vi "MAIN prod-cons combined v1.vi"() -> ()   [LabVIEW 2012]
doc: "Use this template to build a producer/consumer design pattern. Use this template when you need to execute a process, such as data analysis, when a data source, such as a triggered acquisition, produces data at an uneven rate and you need to execute the process when the data becomes available."
uses:
  <vilib>/Instr/_visa.llb/VISA Configure Serial Port (Instr).vi
panel:
  in  "analysis of text file on/off":bool
  in  "stop reading the text file":bool
  in  "INPUT:\non = serial\noff = text file":bool
  in  "XON Character":u8=17 format="%.0x"
  in  "XOFF Character":u8=19 format="%.0x"
  in  "flow control":u16(ring) items=["None"=0, "XON/XOFF"=1, "RTS/CTS"=2, "DTR/DSR"=4]
  in  "End write with termination character?":bool=TRUE
  in  "Input\nbuffer size":u32=4096
  in  "bytes to read":u32=1000
  out "actual bytes read":u32
  in  "write":bool=TRUE
  in  "read":bool=TRUE
  in  "stop 2":bool
  in  "string to write":string="*IDN?"
  in  "termination char\n(0xA = '\\n' = LF)":u8=10 format="%.0x"
  in  "End read on termination character?":bool=TRUE
  in  "timeout (ms)":u32=10000
  in  "stop bits":u16(ring)=10 items=["1.0"=10, "1.5"=15, "2.0"=20]
  in  "parity":u16(ring) items=["None", "Odd", "Even", "Mark", "Space"]
  in  "data bits":u16=8 min=5 max=8 step=1
  in  "VISA resource name":refnum<visa-resource-name>="COM1"
  in  "baud rate":u32=9600
  out "Camera 1":picture
  out "Temperature":waveform(i64)[](graph)
  out "Pressure":waveform(i64)[](graph)
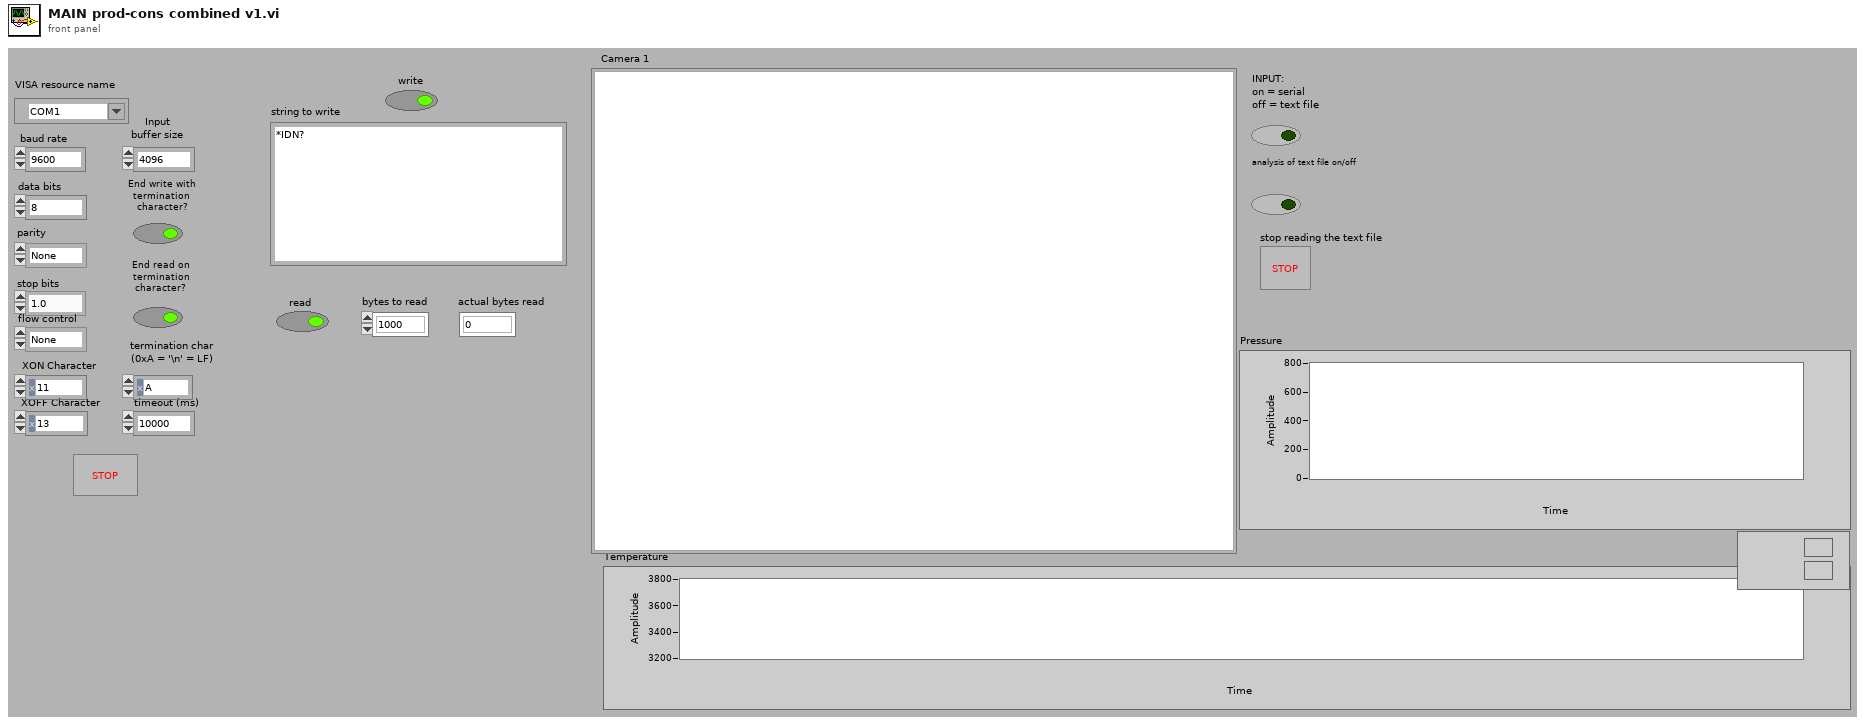
[diagram p1: front panel]
types:
  T1 = enum16{"open", "replace", "create", "open or create", "replace or create", "replace or create with confirmation"}
  T2 = cluster{"left":i16, "top":i16, "right":i16, "bottom":i16}
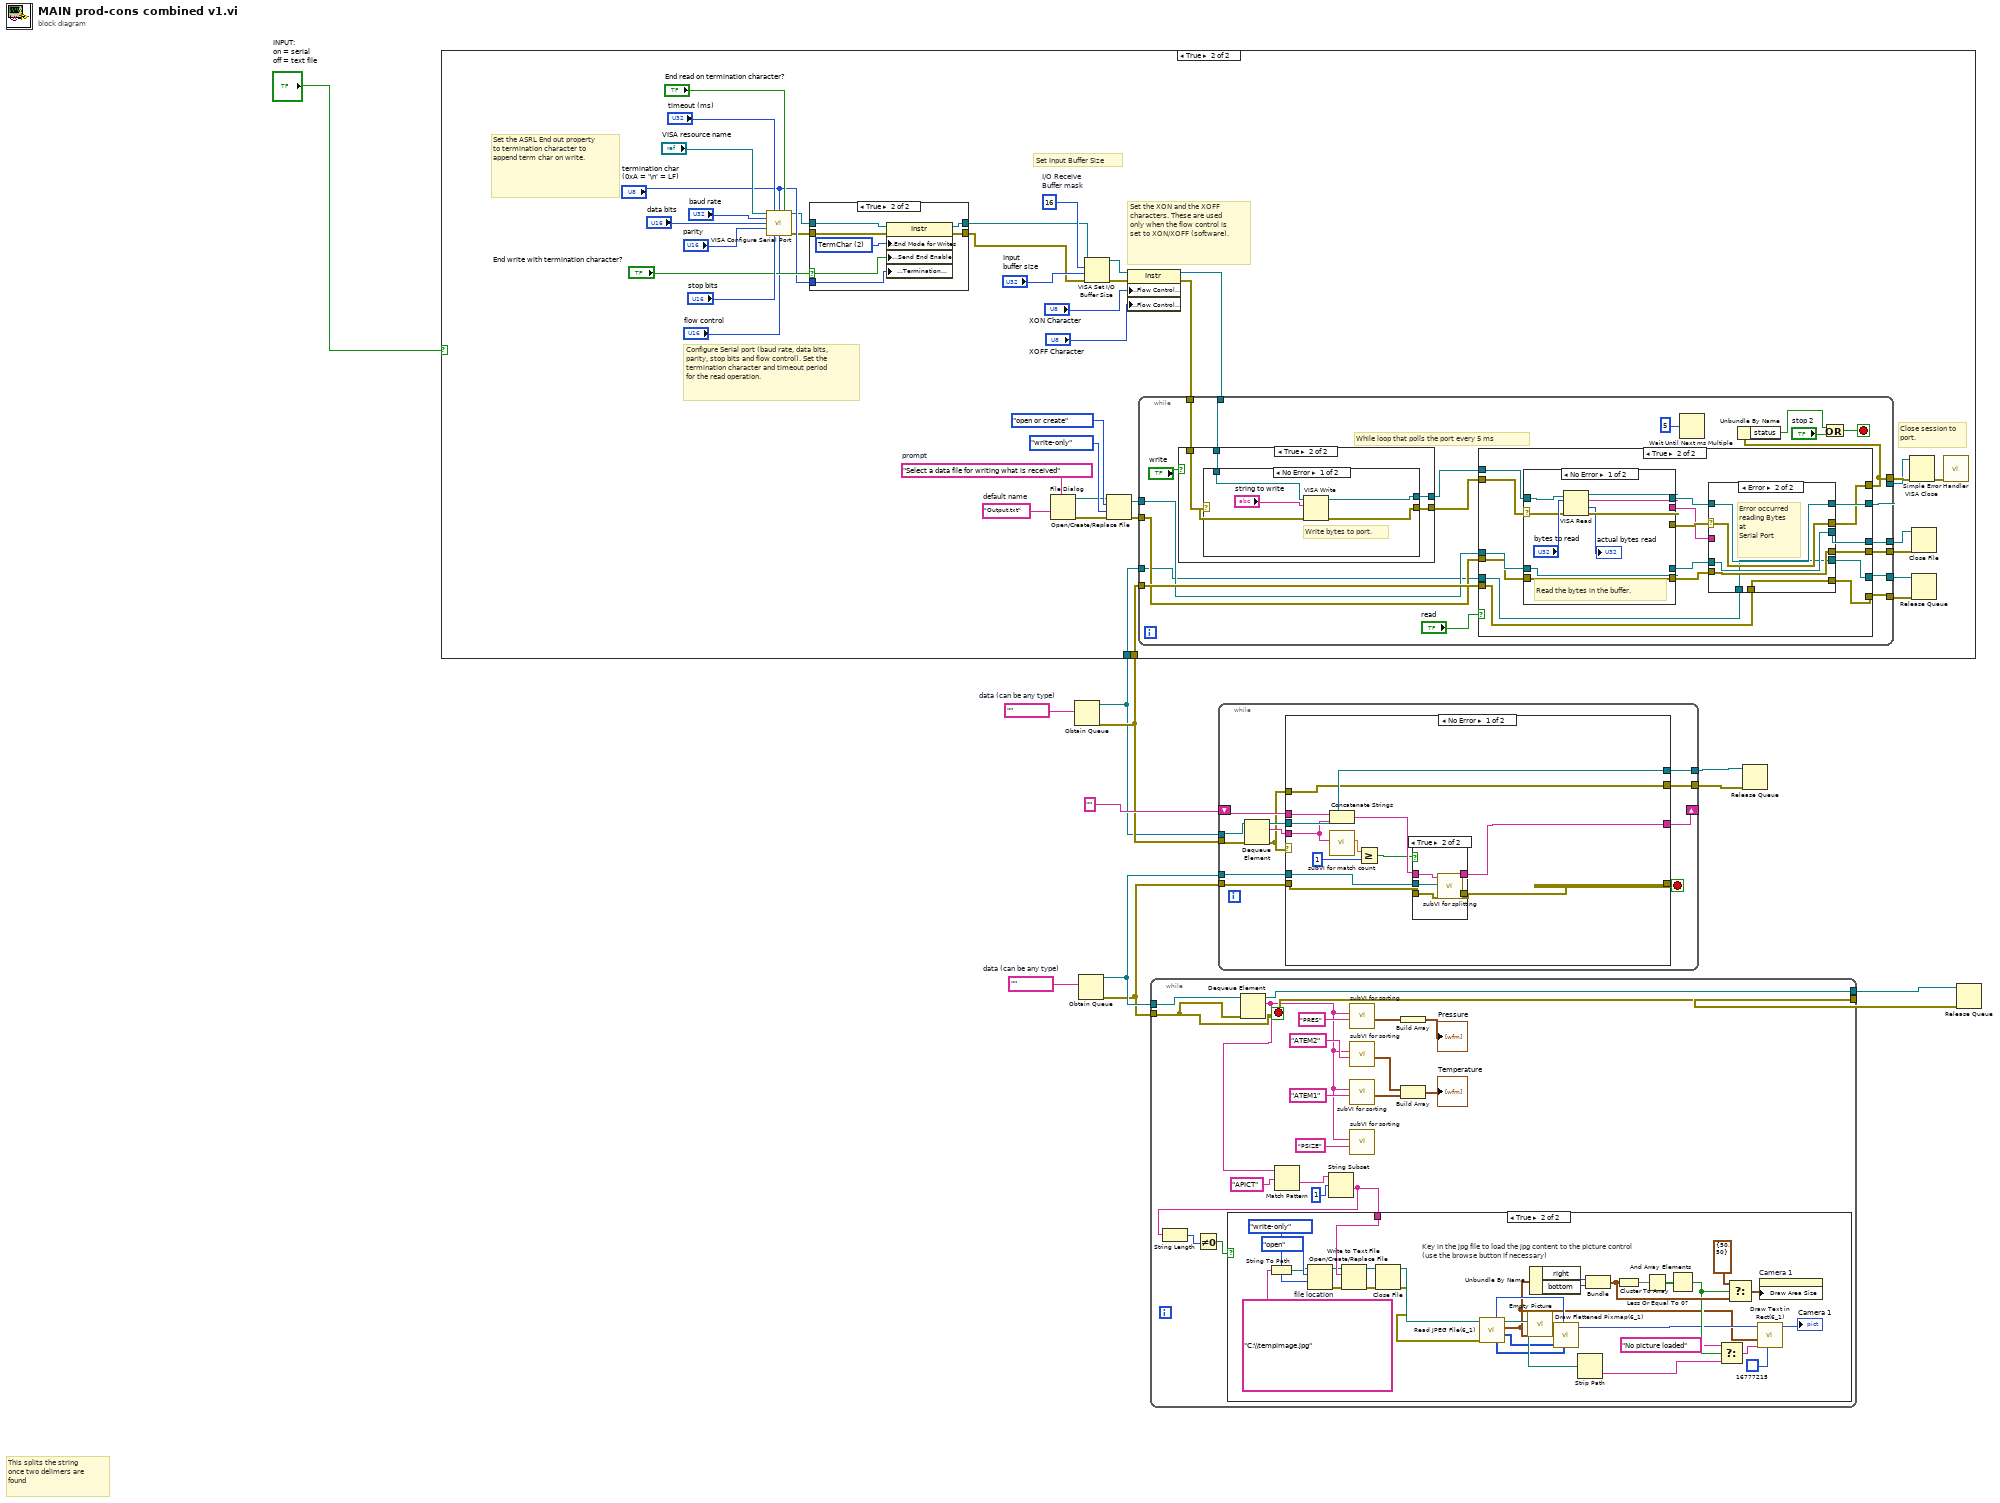
[diagram p0: block diagram]
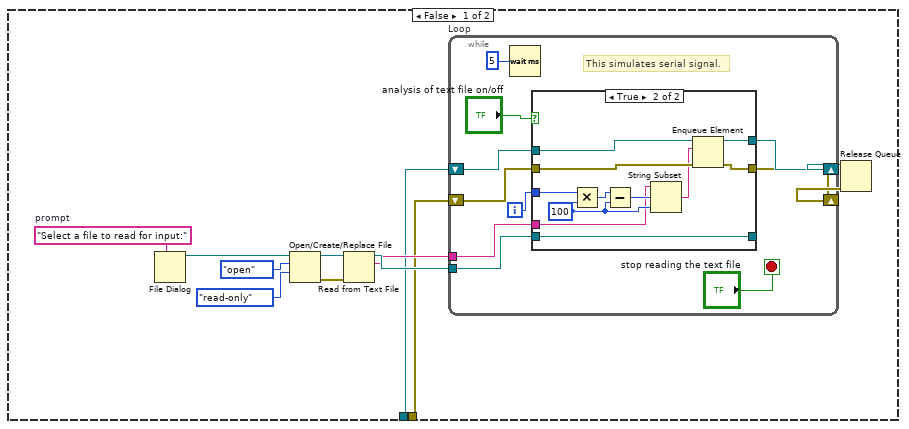
[diagram p2: hidden frame]
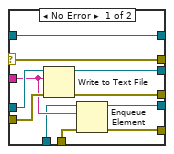
[diagram p8: hidden frame]
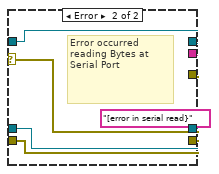
[diagram p9: hidden frame]
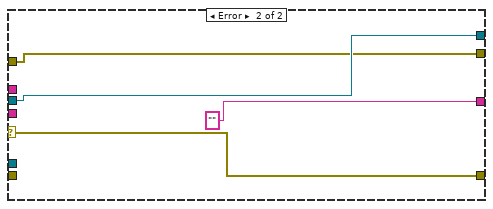
[diagram p12: hidden frame]
diagram:
  w11 = ""  # data (can be any type)
  w12 = ""  # data (can be any type)
  # "This splits the string once two delimers are found"
  n1 = Obtain Queue(element data type=w12) -> (queue out=w2:refnum<queue>, error out=w3:errorcluster)  [unwired: 4 in, 1 out]
  n2 = case shown="True" "INPUT:\non = serial\noff = text file" {
    tunnel: w3 -> [w14 w50]
    tunnel: w2 -> [w13 w49]
    frame False {
      w18 = "Select a file to read for input:"  # prompt
      n3 = File Dialog(7:w18) -> (3:w16:path)  [unwired: 1 in, 8 out]
      n4 = Open/Create/Replace File(file path (use dialog)=w16, operation (0:open)=T1."open", access (0:read/write)=enum16{"read/write", "read-only", "write-only"}."read-only") -> (refnum out=w21:refnum<file>, error out=w22:errorcluster)  [unwired: 1 in, 3 out]
      n5 = Read from Text File(file (use dialog)=w21, error in=w22) -> (refnum out=w17:refnum<file>, text=w15:string)  [unwired: 1 in, 3 out]
      n6 = while "Loop" {
        shift-right: [w26] -> w23
        shift-left: w14 -> [w32]
        shift-right: [w27] -> w24
        shift-left: w13 -> [w33]
        tunnel: w15 -> [w31]
        tunnel: w17 -> [w30]
        i -> [w29]
        stop <- "stop reading the text file" stop-if-true
        # "This simulates serial signal."
        n7 = Wait (ms)(milliseconds to wait=u32 5) -> ()  [unwired: 1 out]
        n8 = case shown="True" "analysis of text file on/off" {
          tunnel: w30 -> [w37 w45]
          tunnel: [w37 w45] -> _
          tunnel: w31 -> [_ w43]
          tunnel: w33 -> [w35 w41]
          tunnel: w32 -> [w36 w40]
          tunnel: w29 -> [_ w44]
          tunnel: [w35 w42] -> w27
          tunnel: [w36 w39] -> w26
          frame False {
          }
          frame True {
            w46 = 100
            n9 = Multiply(x=w44, y=w46) -> (x*y=w48:i32)
            n10 = Subtract(x=w48, y=w46) -> (x-y=w47:i32)
            n11 = String Subset(string=w43, offset (0)=w47, length (rest)=w46) -> (substring=w38:string)
            n12 = Enqueue Element(queue=w41, element=w38, error in (no error)=w40) -> (queue out=w42:refnum<queue>, error out=w39:errorcluster)  [unwired: 1 in, 1 out]
          }
        }
      }
      n13 = Release Queue(queue=w24, error in (no error)=w23) -> ()  [unwired: 1 in, 3 out]
    }
    frame True {
      w59 = "Output.txt"  # default name
      w60 = "Select a data file for writing what is received"  # prompt
      w80 = u16 16  # I/O Receive Buffer mask
      # "Set the XON and the XOFF characters. These are used only when the flow control is set to XON/XOFF (software)."
      # "Configure Serial port (baud rate, data bits, parity, stop bits and flow control). Set the termination character and timeout period for the read operation."
      # "Set Input Buffer Size"
      # "Set the ASRL End out property to termination character to append term char on write."
      # "Close session to port."
      n14 = call-poly "VISA Configure Serial Port"("VISA resource name"="VISA resource name", "timeout (10sec)"="timeout (ms)", "termination char\n(0xA = '\\n' = LF)"="termination char\n(0xA = '\\n' = LF)", "Enable Termination\nChar (T)"="End read on termination character?", "baud rate (9600)"="baud rate", "data bits (8)"="data bits", "parity (0:none)"="parity", "stop bits (10: 1 bit)"="stop bits", "flow control (0:none)"="flow control") -> ("VISA resource name out"=w66:refnum<visa-resource-name>, "error out"=w69:errorcluster)  [unwired: 1 in, 4 out]
      n15 = case shown="True" "End write with termination character?" {
        selector: "End write with termination character?" -> [_ w90]
        tunnel: w66 -> [w88 w96]
        tunnel: w69 -> [w89 w95]
        tunnel: [w88 w94] -> w67
        tunnel: [w89 w93] -> w68
        tunnel: "termination char\n(0xA = '\\n' = LF)" -> [_ w91]
        frame False {
        }
        frame True {
          w92 = u16 2 items=["None", "LastBit", "TermChar", "Break"] ("Serial Settings:Serial End Mode for Writes")
          n16 = property class="Instr"(reference=w96, error in=w95, "Serial Settings:End Mode for Writes"=w92, "Message Based Settings:Send End Enable"=w90, "Message Based Settings:Termination Character"=w91) -> (reference out=w94:refnum<visa-resource-name>, error out=w93:errorcluster)
        }
      }
      n17 = File Dialog(7:w60, 9:w59) -> (0:w61:errorcluster, 3:w58:path)  [unwired: 1 in, 6 out]
      n18 = VISA Set I/O Buffer Size(VISA resource name=w67, mask (16)=w80, size (4096)="Input\nbuffer size", error in (no error)=w68) -> (VISA resource name out=w75:refnum<visa-resource-name>, error out=w74:errorcluster)
      n19 = Open/Create/Replace File(file path (use dialog)=w58, error in=w61, operation (0:open)=T1."open or create", access (0:read/write)=enum16{"read/write", "read-only", "write-only"}."write-only") -> (refnum out=w54:refnum<file>, error out=w55:errorcluster)  [unwired: 3 out]
      n20 = property class="Instr"(reference=w75, error in=w74, "Serial Settings:Flow Control XON Character"="XON Character", "Serial Settings:Flow Control XOFF Character"="XOFF Character") -> (reference out=w65:refnum<visa-resource-name>, error out=w71:errorcluster)
      n21 = while {
        tunnel: w71 -> [w97]
        tunnel: w65 -> [w112]
        tunnel: [w104] -> w51
        tunnel: [w100] -> w64
        tunnel: [w109] -> w57
        tunnel: [w108] -> w56
        tunnel: w55 -> [w103]
        tunnel: w54 -> [w102]
        tunnel: [w107] -> w53
        tunnel: [w106] -> w52
        tunnel: w49 -> [w101]
        tunnel: w50 -> [w105]
        stop <- w111 stop-if-true
        # "While loop that polls the port every 5 ms"
        n22 = case shown="True" "write" {
          tunnel: [w118 w122] -> w99
          tunnel: [w117 w121] -> w98
          tunnel: w112 -> [w118 w120]
          tunnel: w97 -> [w117 w119]
          frame False {
          }
          frame True {
            n23 = case shown="No Error" w119 {
              selector: w119 -> [w123 w129]
              tunnel: [w127 w128] -> w122
              tunnel: [w126 w129] -> w121
              tunnel: w120 -> [w124 w128]
              frame No Error {
                # "Write bytes to port."
                n24 = VISA Write(VISA resource name=w124, write buffer="string to write", error in (no error)=w123) -> (VISA resource name out=w127:refnum<visa-resource-name>, error out=w126:errorcluster)  [unwired: 1 out]
              }
              frame Error {
              }
            }
          }
        }
        n25 = case shown="True" "read" {
          tunnel: w98 -> [w134 w152]
          tunnel: w99 -> [w135 w151]
          tunnel: [w134 w141] -> w100
          tunnel: [w135 w143] -> w104
          tunnel: [w132 w145] -> w109
          tunnel: [w133 w147] -> w108
          tunnel: w102 -> [w133 w150]
          tunnel: w103 -> [w132 w149]
          tunnel: [w130 w138] -> w107
          tunnel: [w131 w139] -> w106
          tunnel: w101 -> [w131 w137]
          tunnel: w105 -> [w130 w136]
          frame False {
          }
          frame True {
            n26 = case "Read bytes from port." shown="No Error" w152 {
              selector: w152 -> [w174 w182]
              tunnel: [w177 w182] -> w142
              tunnel: [w178 w183] -> w144
              tunnel: w151 -> [w175 w183]
              tunnel: [w172 w180] -> w146
              tunnel: [w171 w181] -> w148
              tunnel: w150 -> [w171 w181]
              tunnel: w149 -> [w172 w180]
              tunnel: [w170 "[error in serial read}" ("read buffer")] -> w140
              frame No Error {
                # "Read the bytes in the buffer."
                n27 = VISA Read(VISA resource name=w175, byte count="bytes to read", error in (no error)=w174) -> (VISA resource name out=w178:refnum<visa-resource-name>, read buffer=w170:string, return count=→"actual bytes read":u32, error out=w177:errorcluster)
              }
              frame Error {
                # "Error occurred \nreading Bytes at \nSerial Port"
              }
            }
            n28 = case "Read bytes from port." shown="Error" w142 {
              selector: w142 -> [w163 w166]
              tunnel: [w163 w166] -> w141
              tunnel: w148 -> [w159 w169]
              tunnel: [w158 w169] -> w147
              tunnel: w146 -> [w161 w168]
              tunnel: [w160 w168] -> w145
              tunnel: w144 -> [w162 w167]
              tunnel: [w162 w167] -> w143
              tunnel: w140 -> [w155 _]
              tunnel: [w157 w165] -> w139
              tunnel: [w156 w164] -> w138
              tunnel: w137 -> [w154 w165]
              tunnel: w136 -> [w153 w164]
              frame No Error {
                n29 = Write to Text File(file (use dialog)=w159, text=w155, error in=w161) -> (refnum out=w158:refnum<file>, error out=w160:errorcluster)  [unwired: 1 in, 1 out]
                n30 = Enqueue Element(queue=w154, element=w155, error in (no error)=w153) -> (queue out=w157:refnum<queue>, error out=w156:errorcluster)  [unwired: 1 in, 1 out]
              }
              frame Error {
                # "Error occurred \nreading Bytes at \nSerial Port"
              }
            }
          }
        }
        n31 = Wait Until Next ms Multiple(millisecond multiple=u32 5) -> ()  [unwired: 1 out]
        n32 = Unbundle By Name(w100) -> ("status"=w114:bool)
        n33 = Or(x=w114, y="stop 2") -> (x .or. y?=w111:bool)
      }
      n34 = VISA Close(VISA resource name=w51, error in (no error)=w64) -> (error out=w85:errorcluster)
      n35 = Close File(refnum=w56, error in=w57) -> ()  [unwired: 2 out]
      n36 = Release Queue(queue=w52, error in (no error)=w53) -> ()  [unwired: 1 in, 3 out]
      n37 = call <vilib>:"Simple Error Handler.vi"("error in (no error)"=w85) -> ()  [unwired: 1 in, 8 out]
    }
  }
  n38 = Obtain Queue(element data type=w11) -> (queue out=w10:refnum<queue>, error out=w9:errorcluster)  [unwired: 4 in, 1 out]
  n39 = while {
    tunnel: w10 -> [w202]
    tunnel: w9 -> [w201]
    tunnel: [w192] -> w6
    tunnel: [w191] -> w5
    stop <- w201 stop-if-true
    n40 = Dequeue Element(queue=w202, error in (no error)=w201) -> (queue out=w192:refnum<queue>, element=w190:string, error out=w191:errorcluster)  [unwired: 1 in, 1 out]
    n41 = Match Pattern(string=w190, regular expression="APICT" ("identifier")) -> (after substring=w188:string)  [unwired: 1 in, 3 out]
    n42 = String Subset(string=w188, offset (0)=1) -> (substring=w186:string)  [unwired: 1 in]
    n43 = String Length(string=w186) -> (length=w185:i32)
    n44 = Not Equal To 0?(x=w185) -> (x != 0?=w184:bool)
    n45 = case shown="True" w184 {
      tunnel: w186 -> [_ w234]
      frame False {
      }
      frame True {
        w226 = "C:\\tempimage.jpg"  # file location
        # "Key in the jpg file to load the jpg content to the picture control\n(use the browse button if necessary)"
        n46 = String To Path(string=w226) -> (path=w227:path)
        n47 = Open/Create/Replace File(file path (use dialog)=w227, operation (0:open)=T1."open", access (0:read/write)=enum16{"read/write", "read-only", "write-only"}."write-only") -> (refnum out=w229:refnum<file>, error out=w228:errorcluster)  [unwired: 3 in, 1 out]
        n48 = Write to Text File(file (use dialog)=w229, text=w234, error in=w228) -> (refnum out=w233:refnum<file>, error out=w232:errorcluster)  [unwired: 1 in, 1 out]
        n49 = Close File(refnum=w233, error in=w232) -> (path=w205:path, error out=w204:errorcluster)
        n50 = call <vilib>:"Read JPEG File(6_1).vi"("error in (no error)"=w204, "path to JPEG file"=w205) -> ("flattened image data"=w206:u8[], "rect"=w211:T2, "path"=w213:path, "colorTable"=w210:u32[], "depth"=w225:u8)  [unwired: 4 in, 1 out]
        n51 = call "Empty Picture"() -> ("empty picture"=w224:picture)
        n52 = Unbundle By Name(w211) -> ("right"=w222:i16, "bottom"=w223:i16)
        n53 = call <vilib>:"Draw Flattened Pixmap(6_1).vi"("picture"=w224, "bit depth(8)"=w225, "rect"=w211, "flattened pixmap data"=w206, "color table"=w210) -> ("new picture"=w214:picture)  [unwired: 4 in]
        n54 = Strip Path(path=w213) -> (name=w212:string)  [unwired: 1 out]
        n55 = Bundle("right"=w222, "bottom"=w223) -> (w219:cluster{"right":i16, "bottom":i16})  [unwired: 1 in]
        n56 = Cluster To Array(cluster=w219) -> (array=w221:i16[])
        n57 = Less Or Equal To 0?(x=w221) -> (x <= 0?=w220:bool[])
        n58 = And Array Elements(Boolean array=w220) -> (logical AND=w218:bool)
        n59 = Select(t="No picture loaded", s=w218, f=w212) -> (s? t:f=w216:string)
        n60 = Select(t=cluster{"Width":u32, "Height":u32} {"Width"=50, "Height"=50} ("Draw Area Size"), s=w218, f=w219) -> (s? t:f=w208:cluster{"Width":u32, "Height":u32})
        n61 = call <vilib>:"Draw Text in Rect(6_1).vi"("text color(black)"=u32 16777215, "text"=w216, "rect"=w211, "picture"=w214) -> ("new picture"=→"Camera 1":picture)  [unwired: 7 in]
        n62 = property on="Camera 1" class="Pict"("Draw Area Size"=w208) -> ()  [unwired: 2 in, 2 out]
      }
    }
    n63 = call "subVI for sorting.vi"("identifier"="PRES", "string"=w190) -> ("output"=w199:waveform(i64))  [unwired: 7 in, 2 out]
    n64 = call "subVI for sorting.vi"("identifier"="ATEM2", "string"=w190) -> ("output"=w196:waveform(i64))  [unwired: 7 in, 2 out]
    n65 = call "subVI for sorting.vi"("identifier"="ATEM1", "string"=w190) -> ("output"=w194:waveform(i64))  [unwired: 7 in, 2 out]
    n66 = call "subVI for sorting.vi"("identifier"="PSIZE", "string"=w190) -> ()  [unwired: 7 in, 3 out]
    n67 = Build Array(w199) -> (→"Pressure":waveform(i64)[])
    n68 = Build Array(w196, w194) -> (→"Temperature":waveform(i64)[])
  }
  n69 = while {
    tunnel: w2 -> [w246]
    tunnel: w3 -> [w244]
    shift-right: [w243] -> _
    shift-left: "" ("substring") -> [w242]
    tunnel: w9 -> [w241]
    tunnel: w10 -> [w240]
    tunnel: [w237] -> w8
    tunnel: [w236] -> w7
    stop <- w239 stop-if-true
    n70 = Dequeue Element(queue=w246, error in (no error)=w244) -> (queue out=w238:refnum<queue>, element=w245:string, error out=w235:errorcluster)  [unwired: 1 in, 1 out]
    n71 = case shown="No Error" w235 {
      selector: w235 -> [_ w268]
      tunnel: w245 -> [w248 _]
      tunnel: [w252 ""] -> w243
      tunnel: w242 -> [w250 _]
      tunnel: w241 -> [w257 _]
      tunnel: w240 -> [w256 _]
      tunnel: [w255 w268] -> w239
      tunnel: w238 -> [w254 w267]
      tunnel: [w254 w267] -> w237
      tunnel: w235 -> [w253 w266]
      tunnel: [w253 w266] -> w236
      frame No Error {
        n72 = Concatenate Strings(w250, w248) -> (w258:string)
        n73 = call "subVI for match count.vi"("String"=w248) -> ("Number of matches for \\n"=w247:dbl)  [unwired: 10 in]
        n74 = Greater Or Equal?(x=w247, y=1 ("x")) -> (x >= y?=w249:bool)
        n75 = case shown="True" w249 {
          tunnel: w258 -> [w260 w263]
          tunnel: [w260 w262] -> w252
          tunnel: [w259 w261] -> w255
          tunnel: w257 -> [w259 w265]
          tunnel: w256 -> [_ w264]
          frame False {
          }
          frame True {
            n76 = call "subVI for splitting.vi"("error in (no error)"=w265, "queue"=w264, "input string"=w263) -> ("error out"=w261:errorcluster, "substring"=w262:string)  [unwired: 6 in, 1 out]
          }
        }
      }
      frame Error {
      }
    }
  }
  n77 = Release Queue(queue=w8, error in (no error)=w7) -> ()  [unwired: 1 in, 3 out]
  n78 = Release Queue(queue=w6, error in (no error)=w5) -> ()  [unwired: 1 in, 3 out]
